vi "NetCDFLabviewDemo1.1.vi"(5 "NetCDF File:":path) -> ()   [LabVIEW 2016]
uses:
  DemoSubVIs/XControls/ArrayTree/ArrayTree.xctl
  DemoSubVIs/XControls/PairTable/PairTable.xctl
panel:
  in  "OK":bool
  in  "Tab Control":enum32{"Global ", "Detail"}(tab)
  out "Global Attributes":cluster{"c":string, "l":string}[](xcontrol)
  out "Attributes":cluster{"c":string, "l":string}[](xcontrol)
  out "var tree":T1(xcontrol)
  out "XY":cluster{dbl[], "value":dbl[]}[](graph) caption="H[0] 's graph"
  out "Text Variable":string caption="datetime[0](dump text)"
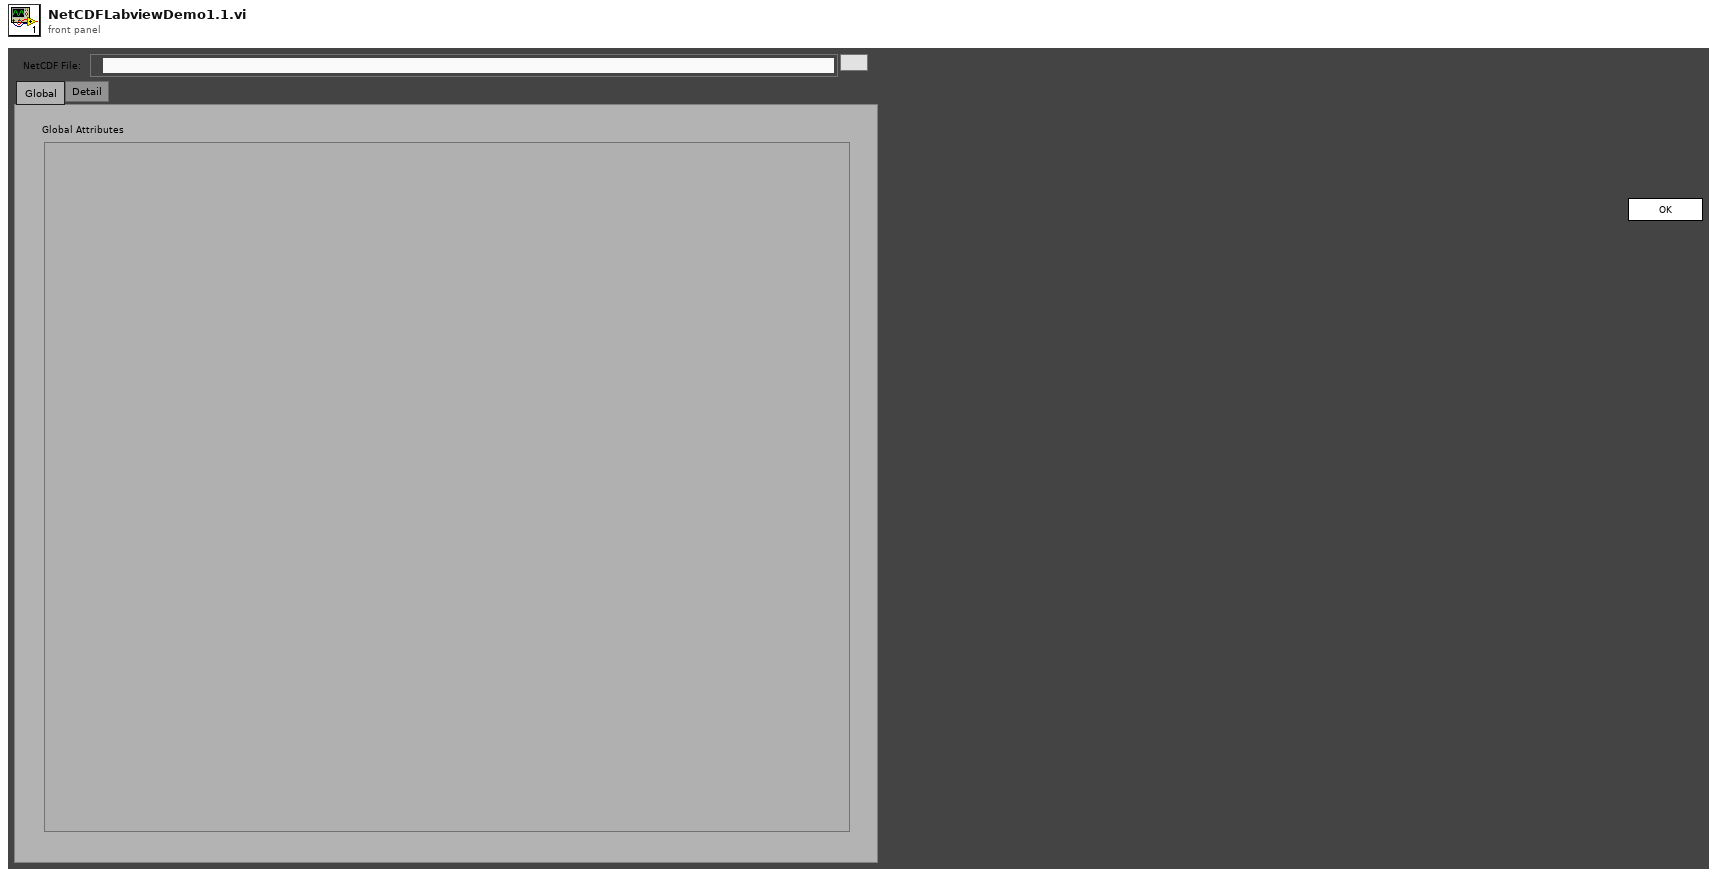
[diagram p1: front panel]
types:
  T1 = cluster{"TopLevelItemName":string, "ChildItemArr":cluster{"ChildDimName":string, "ChildDimSize":u64}[]}[]
  T2 = cluster{"TopLevelItemName":string, "ChildItemArr":cluster{"ChildDimName":string, "ChildDimSize":u64}[]}
  T3 = cluster{"numrecs":u64, "dims":cluster{"name":string, "size":u64}[], "attrs":cluster{"xsz":u64, "name":string, "nc_type":u16, "nelems":u64, "xvalue":string}[], "vars":cluster{"xsz":u64, "shape":u64[], "dsizes":u64[], "name":string, "dimids":u64[], "NC_attrarray":cluster{"xsz":u64, "name":string, "nc_type":u16, "nelems":u64, "xvalue":string}[], "nc_type":enum16{"NC_NAT", "NC_BYTE", "NC_CHAR", "NC_SHORT", "NC_INT", "NC_FLOAT", "NC_DOUBLE"}, "len":u64, "begin":u64}[]}
  T4 = cluster{"xsz":u64, "shape":u64[], "dsizes":u64[], "name":string, "dimids":u64[], "NC_attrarray":cluster{"xsz":u64, "name":string, "nc_type":u16, "nelems":u64, "xvalue":string}[], "nc_type":enum16{"NC_NAT", "NC_BYTE", "NC_CHAR", "NC_SHORT", "NC_INT", "NC_FLOAT", "NC_DOUBLE"}, "len":u64, "begin":u64}[]
  T5 = cluster{"xsz":u64, "shape":u64[], "dsizes":u64[], "name":string, "dimids":u64[], "NC_attrarray":cluster{"xsz":u64, "name":string, "nc_type":u16, "nelems":u64, "xvalue":string}[], "nc_type":enum16{"NC_NAT", "NC_BYTE", "NC_CHAR", "NC_SHORT", "NC_INT", "NC_FLOAT", "NC_DOUBLE"}, "len":u64, "begin":u64}
  T6 = enum32{"Invalid", "Standard", "Closed", "Hidden", "Minimized", "Maximized"}
  T7 = enum32{"invalid app kind", "Development System", "Run Time System", "Student Edition", "Embedded LabVIEW", "Evaluation", "Custom"}
  T8 = cluster{"Core":cluster{"Current VI Reference":refnum<vi>, "Close Panel on Exit?":bool}, "File Path":path, "file reference":refnum<k0>, "VarIndexArr":cluster{"TopLevelItemName":string, "ChildItemArr":cluster{"ChildDimName":string, "ChildDimSize":u64}[]}, "NC":cluster{"numrecs":u64, "dims":cluster{"name":string, "size":u64}[], "attrs":cluster{"xsz":u64, "name":string, "nc_type":u16, "nelems":u64, "xvalue":string}[], "vars":cluster{"xsz":u64, "shape":u64[], "dsizes":u64[], "name":string, "dimids":u64[], "NC_attrarray":cluster{"xsz":u64, "name":string, "nc_type":u16, "nelems":u64, "xvalue":string}[], "nc_type":enum16{"NC_NAT", "NC_BYTE", "NC_CHAR", "NC_SHORT", "NC_INT", "NC_FLOAT", "NC_DOUBLE"}, "len":u64, "begin":u64}[]}, "var-lowest-dim name pair":cluster{"name":string, "name":string}[]}
  T9 = cluster{"Current VI Reference":refnum<vi>, "Close Panel on Exit?":bool}
  T10 = cluster{"xsz":u64, "name":string, "nc_type":u16, "nelems":u64, "xvalue":string}[]
  T11 = cluster{"name":string, cluster{"name":string, "数值":u64}[]}[]
  T12 = enum16{"NC_NAT", "NC_BYTE", "NC_CHAR", "NC_SHORT", "NC_INT", "NC_FLOAT", "NC_DOUBLE"}
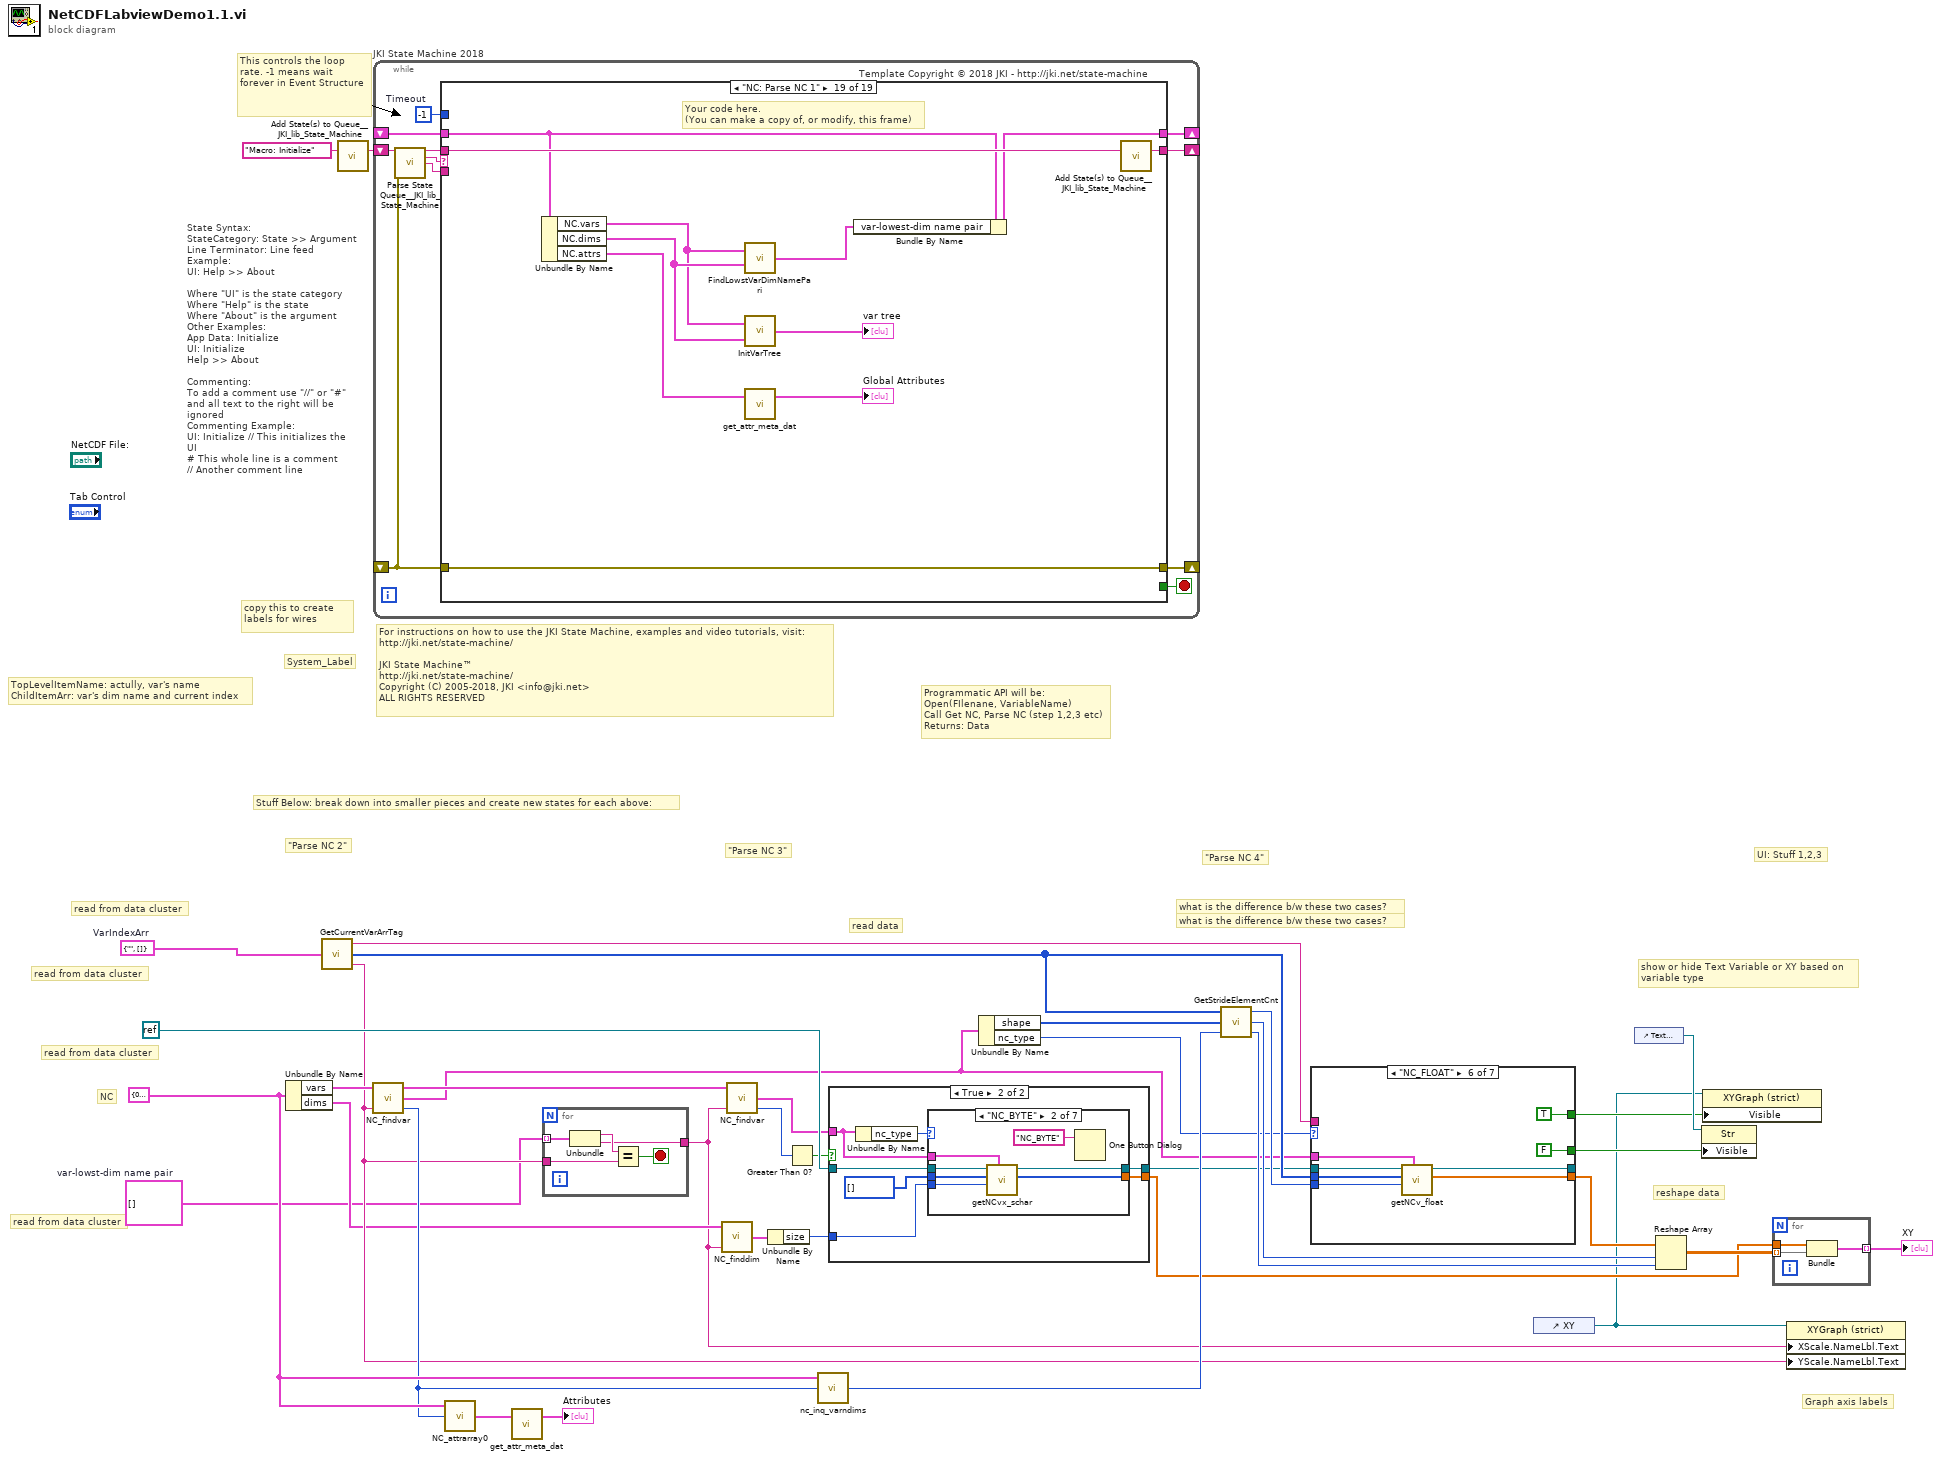
[diagram p0: block diagram]
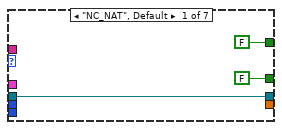
[diagram p2: hidden frame]
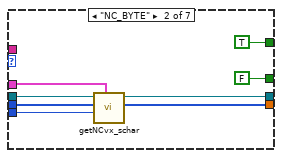
[diagram p3: hidden frame]
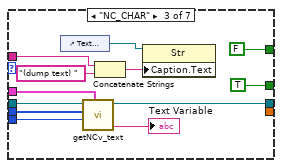
[diagram p4: hidden frame]
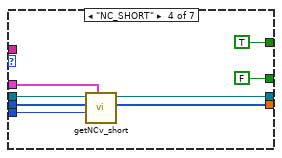
[diagram p5: hidden frame]
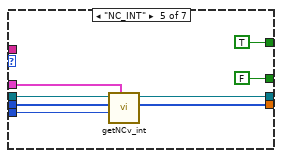
[diagram p6: hidden frame]
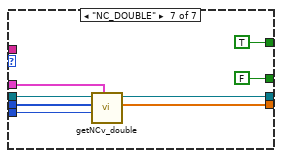
[diagram p7: hidden frame]
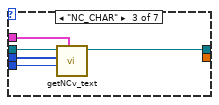
[diagram p10: hidden frame]
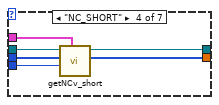
[diagram p11: hidden frame]
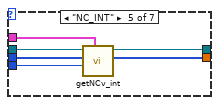
[diagram p12: hidden frame]
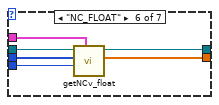
[diagram p13: hidden frame]
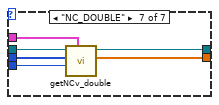
[diagram p14: hidden frame]
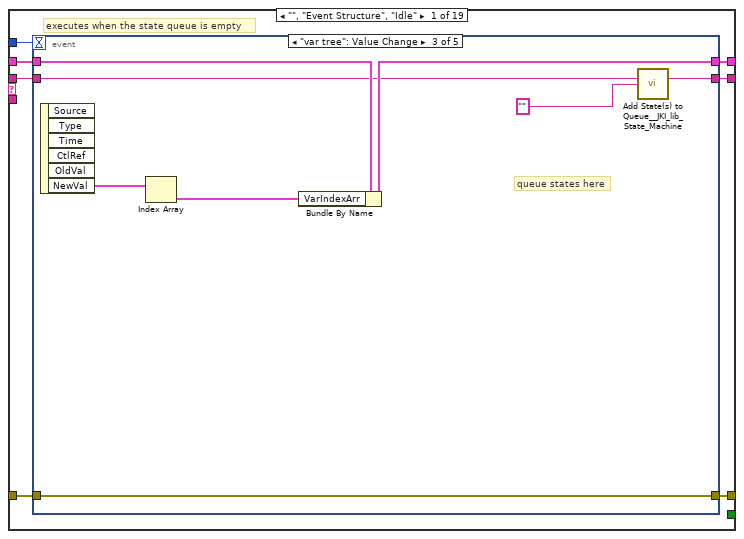
[diagram p15: hidden frame]
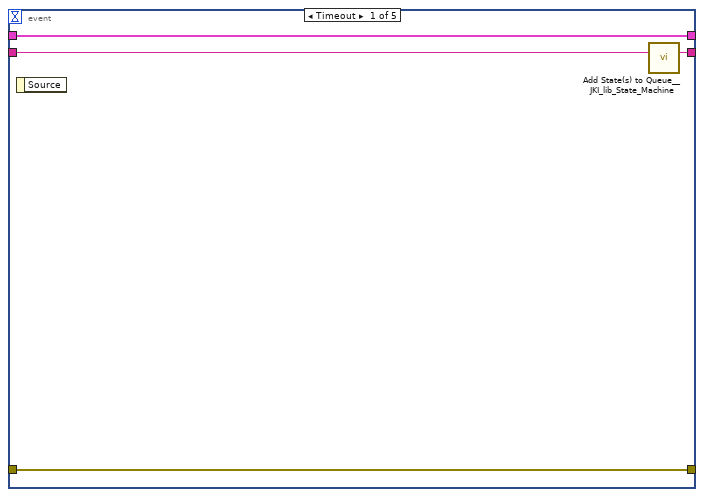
[diagram p16: hidden frame]
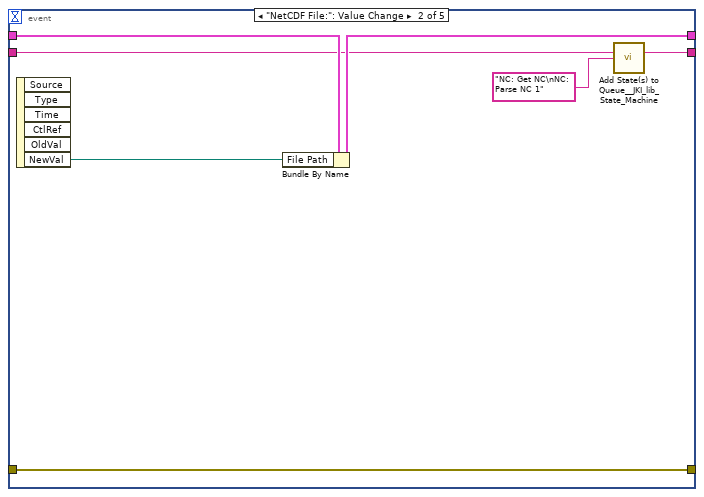
[diagram p17: hidden frame]
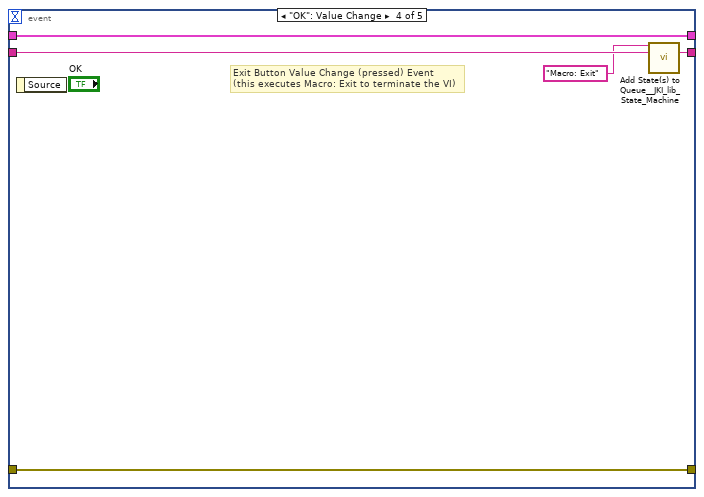
[diagram p18: hidden frame]
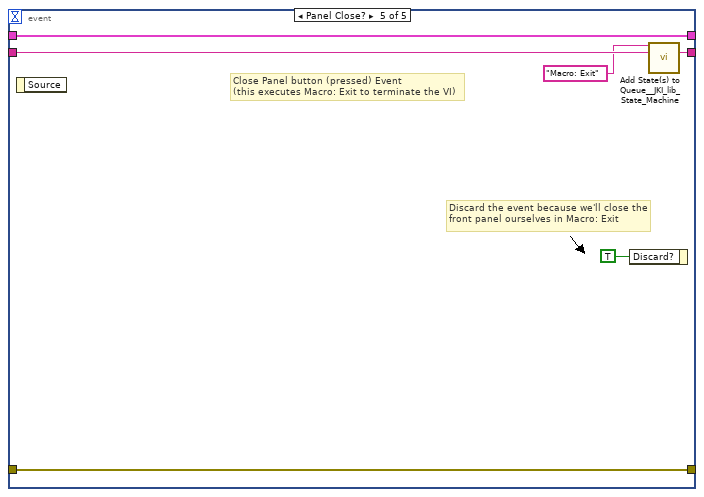
[diagram p19: hidden frame]
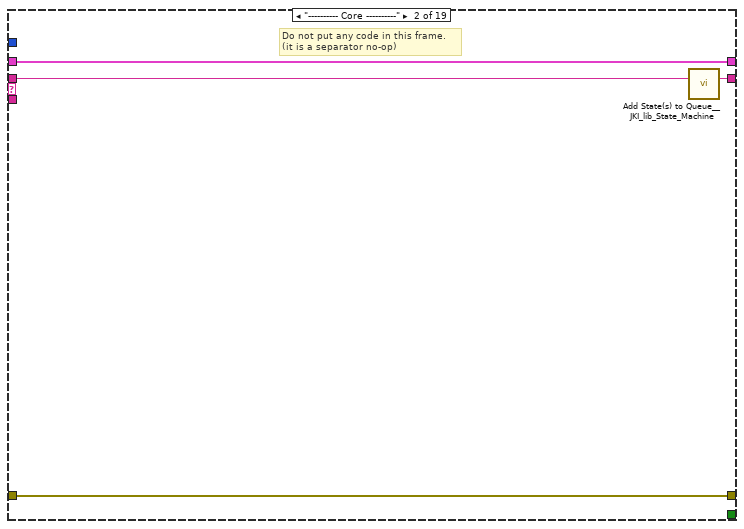
[diagram p20: hidden frame]
diagram:
  w4 = T2 {"TopLevelItemName"="", "ChildItemArr"=[]}  # VarIndexArr
  w2 = cluster{"name":string, "name":string}[] []  # var-lowst-dim name pair
  w34 = T3 {"numrecs"=0, "dims"=[], "attrs"=[], "vars"=[]} ("NC")
  # "Stuff Below: break down into smaller pieces and create new states for each above:"
  # "\"Parse NC 4\""
  # "\"Parse NC 3\""
  # "read from data cluster"
  # "read from data cluster"
  # "read data"
  # "Graph axis labels"
  # "UI: Stuff 1,2,3"
  # "\"Parse NC 2\""
  # "what is the difference b/w these two cases?"
  # "what is the difference b/w these two cases?"
  # "reshape data"
  # "show or hide Text Variable or XY based on\nvariable type"
  # "read from data cluster"
  # "read from data cluster"
  # "Programmatic API will be:\nOpen(FIlenane, VariableName)\nCall Get NC, Parse NC (step 1,2,3 etc)\nReturns: Data"
  # "For instructions on how to use the JKI State Machine, examples and video tutorials, visit:\nhttp://jki.net/state-machine/\n\nJKI State Machine™\nhttp://jki.net/state-machine/\nCopyright (C) 2005-2018, JKI <info@jki.net>\nALL RIGHTS RESERVED"
  # "State Syntax:\nStateCategory: State >> Argument\nLine Terminator: Line feed\nExample:\nUI: Help >> About\n\nWhere \"UI\" is the state category\nWhere \"Help\" is the state\nWhere \"About\" is the argument\nOther Examples:\nApp Data: Initialize\nUI: Initialize\nHelp >> About\n\nCommenting:\nTo add a comment use \"//\" or \"#\" and all text to the right will be ignored\nCommenting Example:\nUI: Initialize // This initializes the UI\n# This whole line is a comment\n// Another comment line"
  # "copy this to create labels for wires"
  # "This controls the loop rate. -1 means wait forever in Event Structure"
  # "System_Label"
  # "TopLevelItemName: actully, var's name\nChildItemArr: var's dim name and current index"
  # "NC"
  n1 = Unbundle By Name(w34) -> ("vars"=w14:T4, "dims"=w11:cluster{"name":string, "size":u64}[])
  n2 = call "GetCurrentVarArrTag.vi"("VarIndexArr"=w4) -> ("CurrentArrayTag"=w16:string, "IndexTagArr"=w18:u64[], "TopLevelItemName"=w13:string)
  n3 = call <vilib>:"Add State(s) to Queue__JKI_lib_State_Machine.vi"("State(s) in (\"\")"="Macro: Initialize") -> ("States Out"=w36:string)  [unwired: 14 in]
  n4 = call "NC_findvar.vi"("name"=w13, "NC_vararray"=w14) -> ("varid"=w29:i32, "NC_var"=w9:T5, "NC_vararray  out"=w12:T4)  [unwired: 1 out]
  n5 = while "JKI State Machine 2018" {
    shift-right: [w41] -> _
    shift-left: _ -> [w40]
    shift-right: [w44] -> _
    shift-left: _ -> [w38]
    shift-right: [w43] -> _
    shift-left: w36 -> [w45]
    stop <- w42 stop-if-true
    w39 = -1  # Timeout
    # "Template Copyright © 2018 JKI - http://jki.net/state-machine"
    n6 = call <vilib>:"Parse State Queue__JKI_lib_State_Machine.vi"("State Queue"=w45, "Error In (no error)"=w38) -> ("Remaining States"=w47:string, "Current State"=w48:string, "Arguments"=w46:string)  [unwired: 11 in]
    n7 = case shown="\"NC: Parse NC 1\"" w48 {
      selector: w48 -> [_ _ w90 _ _ _ _ _ _ _ _ _ _ _ _ _ _ _ _]
      tunnel: w47 -> [w55 w89 w94 w113 w119 w124 w128 w138 w146 w150 w154 w160 w171 w240 w245 w255 w259 w268 w279]
      tunnel: w46 -> [_ _ _ _ _ _ _ _ _ _ _ w155 w165 _ _ _ _ _ _]
      tunnel: w40 -> [w53 w86 w92 w106 w116 w122 w125 _ w142 w147 w152 w158 w167 w237 w242 w252 w256 w261 w270]
      tunnel: [w52 w87 w96 w110 errorcluster {"status"=FALSE, "code"=0, "source"=""} ("error out") w121 w126 w135 w143 w148 w151 w156 w168 w238 w243 w253 w257 w264 w277] -> w44
      tunnel: w38 -> [w51 w87 w95 w110 w115 w121 w126 w135 w140 w148 w151 w157 w169 w238 w243 w253 w257 w265 w277]
      tunnel: [w54 w88 w93 w112 w118 w123 w127 w137 w145 w149 w153 w159 w170 w239 w244 w254 w258 w267 w278] -> w43
      tunnel: [_ _ _ _ _ TRUE _ _ _ _ _ _ _ _ _ _ _ _ _] -> w42
      tunnel: [w50 w86 w92 w111 w116 w122 w125 w136 w142 w147 w152 w158 w167 w237 w242 w252 w256 w260 w269] -> w41
      tunnel: w39 -> [w49 _ _ _ _ _ _ _ _ _ _ _ _ _ _ _ _ _ _]
      frame "", "Event Structure", "Idle" {
        # "executes when the state queue is empty"
        n8 = event shown="[2] \"var tree\": Value Change" {
          selector: _ -> [_ _ _ _ _]
          dyn-events: _ -> [_ _ _ _ _]
          timeout: w49 -> [_ _ _ _ _]
          tunnel: w55 -> [w59 w61 w70 w79 w85]
          tunnel: [w58 w60 w69 w78 w84] -> w54
          tunnel: w53 -> [w56 w65 w73 w76 w82]
          tunnel: [w57 w66 w74 w77 w83] -> w52
          tunnel: w51 -> [w57 w66 w74 w77 w83]
          tunnel: [w56 w64 w72 w76 w82] -> w50
          event Timeout {
            n9 = event-data() -> ()  [unwired: 1 in, 1 out]
            n10 = call <vilib>:"Add State(s) to Queue__JKI_lib_State_Machine.vi"("State(s) in (\"\")"=w59) -> ("States Out"=w58:string)  [unwired: 14 in]
          }
          event "NetCDF File:": Value Change {
            n11 = event-data() -> ("NewVal"=w63:path)  [unwired: 1 in, 5 out]
            n12 = Bundle By Name(cluster=w65, "File Path"=w63) -> (w64:T8)
            n13 = call <vilib>:"Add State(s) to Queue__JKI_lib_State_Machine.vi"("State(s) in (\"\")"=w61, "State(s) at Back (\"\")"="NC: Get NC\nNC: Parse NC 1" ("State(s) at Back (\"\")")) -> ("States Out"=w60:string)  [unwired: 13 in]
          }
          event "var tree": Value Change {
            # "queue states here"
            n14 = event-data() -> ("NewVal"=w68:T1)  [unwired: 1 in, 5 out]
            n15 = Index Array(array=w68) -> (element=w67:T2)  [unwired: 1 in]
            n16 = Bundle By Name(cluster=w73, "VarIndexArr"=w67) -> (w72:T8)
            n17 = call <vilib>:"Add State(s) to Queue__JKI_lib_State_Machine.vi"("State(s) in (\"\")"=w70, "State(s) at Back (\"\")"="" ("State(s) at Back (\"\")")) -> ("States Out"=w69:string)  [unwired: 13 in]
          }
          event "OK": Value Change {
            # "Exit Button Value Change (pressed) Event\n(this executes Macro: Exit to terminate the VI)"
            n18 = event-data() -> ()  [unwired: 1 in, 1 out]
            n19 = call <vilib>:"Add State(s) to Queue__JKI_lib_State_Machine.vi"("State(s) in Front (\"\")"="Macro: Exit", "State(s) in (\"\")"=w79) -> ("States Out"=w78:string)  [unwired: 13 in]
          }
          event Panel Close? {
            # "Discard the event because we'll close the front panel ourselves in Macro: Exit"
            # "Close Panel button (pressed) Event\n(this executes Macro: Exit to terminate the VI)"
            n20 = event-data() -> ()  [unwired: 1 in, 1 out]
            n21 = event-data("Discard?"=TRUE) -> ()  [unwired: 1 in, 1 out]
            n22 = call <vilib>:"Add State(s) to Queue__JKI_lib_State_Machine.vi"("State(s) in Front (\"\")"="Macro: Exit", "State(s) in (\"\")"=w85) -> ("States Out"=w84:string)  [unwired: 13 in]
          }
        }
      }
      frame "---------- Core ----------" {
        # "Do not put any code in this frame.\n(it is a separator no-op)"
        n23 = call <vilib>:"Add State(s) to Queue__JKI_lib_State_Machine.vi"("State(s) in (\"\")"=w89) -> ("States Out"=w88:string)  [unwired: 14 in]
      }
      frame Default {
        w99 = 42 items=["No error", "Argument error", "Memory is full", "Out of zone", "End of file", "File already open", "Generic file I/O error", "File not found", "File permission error", "Disk is full", "Duplicate path", "Too many files open", "System feature not enabled", "Resource file not found", "Cannot add resource", "Resource not found", "Image not found", "Image memory error", "Pen does not exist", "Config type invalid", "Config token not found", "Config parse error", "Config memory error", "Bad external code format", "Bad external code offset", "External code not present", "Null window", "Destroy window error", "Null menu", "Print aborted", "Bad print record", "Print driver error", "Windows error during printing", "Memory error during printing", "Print dialog error", "Generic print error", "Invalid device refnum", "Device not found", "Device parameter error", "Device unit error", "Cannot open device", "Device call aborted", "Generic error", "Cancelled by user", "Object ID too low", "Object ID too high", "Object not in heap", "Unknown heap", "Unknown object (invalid DefProc)", "Unknown object (DefProc not in table)", "Message out of range", "Invalid (null) method", "Unknown message", "Manager call not supported", "Bad address", "Network operation in progress", "Network operation timed out", "Connection is busy", "Network attribute not supported", "Network error", "Address in use", "System out of memory", "Connection aborted", "Connection refused", "Not connected", "Already connected", "Connection closed", "Initialization error (interapplication manager)", "Bad occurrence", "Wait on unbound occurrence handler", "Occurrence queue overflow", "Datalog type conflict", "Unused", "Unrecognized type (interapplication manager)", "Memory corrupt", "Failed to make temporary DLL", "Old CIN version", "Drag socket not found", "Failed to load drop-object", "Failed to register OLE object", "Failed to release OLE object", "Format specifier type mismatch", "Unknown format specifier", "Too few format specifiers", "Too many format specifiers", "Scan failed", "Newer CIN version", "Error converting to variant", "Runtime menu error", "Password tampered", "Variant attribute not found", "Incompatible variant data type", "Event data is not available", "Event Store is not present", "Occurrence is not found", "Event Queue is not created", "Event info is not available", "Refnum passed is NULL", "Error retrieving Class GUID", "Error retrieving CoClass GUID", "Error retrieving TypeLib GUID.", "Bad built application magic bytes.", "Specific driver is different from the specific driver associated with the Logical Name.", "There is no session opened to the class driver.", "Max Error", "MAX - Error with config objects", "MAX - Error loading configuration", "MAX - Group not supported"]
        # "Current State"
        # "Do not delete, rename, or modify this frame.\n(this is used to capture unhandled states and typos)"
        # "Handle mistyped state name (developer tool)"
        n24 = Format Into String(format string="Software Exception: Unhandled State \"%s\"." ("message"), error in=w95, w90) -> (resulting string=w98:string, error out=w97:errorcluster)  [unwired: 1 in]
        n25 = call <vilib>:"Error Cluster From Error Code.vi"("show call chain? (False)"=TRUE, "error in (no error)"=w97, "error message (\"\")"=w98, "error code (0)"=w99) -> ("error out"=w96:errorcluster)  [unwired: 5 in]
        n26 = call <vilib>:"Add State(s) to Queue__JKI_lib_State_Machine.vi"("State(s) in (\"\")"=w94) -> ("States Out"=w93:string)  [unwired: 14 in]
      }
      frame "Initialize Core Data" {
        # "Do not delete, rename, or modify this frame.\n(this is used to determine panel behavior on exit)"
        # "originally closed?"
        # "exe?"
        # "If panel starts closed or is an EXE, then close it when we exit"
        n27 = property class="VI"() -> ("FP.State"=w103:T6)  [unwired: 2 in, 2 out]
        n28 = property class="App"() -> ("App.Kind"=w109:T7)  [unwired: 2 in, 2 out]
        n29 = control-ref of="Current VI Reference"() -> (w104:refnum<vi>)
        n30 = Equal?(x=w103, y=T6."Closed" ("Front Panel Window:State")) -> (x = y?=w101:bool)
        n31 = Equal?(x=w109, y=T7."Run Time System" ("Application:Kind")) -> (x = y?=w107:bool)
        n32 = Or(x=w101, y=w107) -> (x .or. y?=w105:bool)
        n33 = Bundle By Name(cluster=w106, "Core.Current VI Reference"=w104, "Core.Close Panel on Exit?"=w105) -> (w111:T8)
        n34 = call <vilib>:"Add State(s) to Queue__JKI_lib_State_Machine.vi"("State(s) in (\"\")"=w113) -> ("States Out"=w112:string)  [unwired: 14 in]
      }
      frame "Error Handler" {
        # "Unhandled Error -- Display it"
        # "Handle any errors here.\nYou can also output any states to clean-up after errors occur"
        # "Clear error"
        n35 = call <vilib>:"General Error Handler.vi"("error in (no error)"=w115) -> ()  [unwired: 10 in, 5 out]
        n36 = call <vilib>:"Add State(s) to Queue__JKI_lib_State_Machine.vi"("State(s) in Front (\"\")"="/* Post Error States", "State(s) in (\"\")"=w119) -> ("States Out"=w118:string)  [unwired: 13 in]
      }
      frame "Exit" {
        # "Do not put any code in this frame.\n(No errors that occur here will be handled.)"
        n37 = call <vilib>:"Add State(s) to Queue__JKI_lib_State_Machine.vi"("State(s) in (\"\")"=w124) -> ("States Out"=w123:string)  [unwired: 14 in]
      }
      frame "---------- Data ----------" {
        # "Do not put any code in this frame.\n(It is a separator no-op. You can make a copy of this frame to create a new Data frame)"
        n38 = call <vilib>:"Add State(s) to Queue__JKI_lib_State_Machine.vi"("State(s) in (\"\")"=w128) -> ("States Out"=w127:string)  [unwired: 14 in]
      }
      frame "Data: Initialize" {
        w129 = T2 {"TopLevelItemName"="", "ChildItemArr"=[]}  # VarIndexArr
        w130 = cluster{"name":string, "name":string}[] []  # var-lowest-dim name pair
        w131 = refnum<k0> refnum  # file reference
        w132 = path ""  # File Path
        w133 = T3 {"numrecs"=0, "dims"=[], "attrs"=[], "vars"=[]}  # NC
        w134 = T9 {"Current VI Reference"=refnum, "Close Panel on Exit?"=FALSE}  # Core
        # "Initialize the shift-register data, here.\n(data names are defined by what you wire into the bundle function)"
        n39 = Bundle("Core"=w134, "File Path"=w132, "file reference"=w131, "VarIndexArr"=w129, "NC"=w133, "var-lowest-dim name pair"=w130) -> (w136:T8)  [unwired: 1 in]
        n40 = call <vilib>:"Add State(s) to Queue__JKI_lib_State_Machine.vi"("State(s) in (\"\")"=w138) -> ("States Out"=w137:string)  [unwired: 14 in]
      }
      frame "Data: Cleanup" {
        # "Cleanup any data and references, here.\n(this is called automatically, by the Macro: Exit)"
        n41 = Unbundle By Name(w142) -> ("Core.Current VI Reference"=w144:refnum<vi>, "file reference"=w141:refnum<k0>)
        n42 = Close File(refnum=w141, error in=w140) -> (error out=w139:errorcluster)  [unwired: 1 out]
        n43 = Close Reference(reference=w144, error in (no error)=w139) -> (error out=w143:errorcluster)
        n44 = call <vilib>:"Add State(s) to Queue__JKI_lib_State_Machine.vi"("State(s) in (\"\")"=w146) -> ("States Out"=w145:string)  [unwired: 14 in]
      }
      frame "---------- UI ----------" {
        # "Do not put any code in this frame.\n(It is a separator no-op. You can make a copy of this frame to create a new UI frame)"
        n45 = call <vilib>:"Add State(s) to Queue__JKI_lib_State_Machine.vi"("State(s) in (\"\")"=w150) -> ("States Out"=w149:string)  [unwired: 14 in]
      }
      frame "UI: Initialize" {
        # "Initialize the User Interface, here.\n(this is called automatically, by the Macro: Init)"
        n46 = call <vilib>:"Add State(s) to Queue__JKI_lib_State_Machine.vi"("State(s) in (\"\")"=w154) -> ("States Out"=w153:string)  [unwired: 14 in]
      }
      frame "UI: Cursor Set" {
        # "Argument"
        # "Set and Unset Cursor Busy.\n(Usage: \"UI: Cursor Set >> Busy|Idle\")"
        n47 = case shown="\"Idle\", Default" w155 {
          tunnel: w157 -> [w162 w164]
          tunnel: [w161 w163] -> w156
          frame "Idle", Default {
            n48 = call <vilib>:"Unset Busy.vi"("error in (no error)"=w162) -> ("error out"=w161:errorcluster)  [unwired: 10 in]
          }
          frame "Busy" {
            n49 = call <vilib>:"Set Busy.vi"("error in (no error)"=w164) -> ("error out"=w163:errorcluster)  [unwired: 9 in, 1 out]
          }
        }
        n50 = call <vilib>:"Add State(s) to Queue__JKI_lib_State_Machine.vi"("State(s) in (\"\")"=w160) -> ("States Out"=w159:string)  [unwired: 14 in]
      }
      frame "UI: Front Panel State" {
        # "Argument"
        # "Set Front Panel Open or Closed\n(Usage: \"UI: Front Panel State >> Open|Close\")"
        n51 = Unbundle By Name(w167) -> ("Core.Current VI Reference"=w166:refnum<vi>)
        n52 = case shown="\"Minimize\", \"Minimized\"" w165 {
          tunnel: w169 -> [w177 w192 w203 w216 w229]
          tunnel: [w179 w193 w205 w218 w231] -> w168
          tunnel: w166 -> [w178 w190 w204 w217 w230]
          frame "Open", "Standard", Default {
            w172 = T6."Standard" ("State")
            n53 = property class="VI"(reference=w178, error in=w177) -> (reference out=w175:refnum<vi>, error out=w176:errorcluster, "FP.State"=w174:T6)
            n54 = Not Equal?(x=w174, y=w172) -> (x != y?=w173:bool)
            n55 = case shown="True" w173 {
              tunnel: [w183 w185] -> w179
              tunnel: w176 -> [w182 w185]
              tunnel: w175 -> [w181 _]
              tunnel: w172 -> [w180 _]
              frame True {
                n56 = invoke class="VI" method="FP.Open"(reference=w181, error in=w182, "Activate"=TRUE, "State"=w180) -> (error out=w183:errorcluster)  [unwired: 1 in, 4 out]
              }
              frame False {
              }
            }
          }
          frame "Close", "Closed" {
            n57 = property class="VI"(reference=w190, error in=w192) -> (reference out=w189:refnum<vi>, error out=w191:errorcluster, "FP.State"=w187:T6)
            n58 = Not Equal?(x=w187, y=T6."Closed" ("Front Panel Window:State")) -> (x != y?=w186:bool)
            n59 = case shown="True" w186 {
              tunnel: [w194 w197] -> w193
              tunnel: w191 -> [w194 w196]
              tunnel: w189 -> [_ w195]
              frame False {
              }
              frame True {
                n60 = invoke class="VI" method="FP.Close"(reference=w195, error in=w196) -> (error out=w197:errorcluster)  [unwired: 1 in, 2 out]
              }
            }
          }
          frame "Hidden", "Hide" {
            w198 = T6."Hidden" ("State")
            n61 = property class="VI"(reference=w204, error in=w203) -> (reference out=w201:refnum<vi>, error out=w202:errorcluster, "FP.State"=w200:T6)
            n62 = Not Equal?(x=w200, y=w198) -> (x != y?=w199:bool)
            n63 = case shown="True" w199 {
              tunnel: [w209 w210] -> w205
              tunnel: w202 -> [w208 w210]
              tunnel: w201 -> [w207 _]
              tunnel: w198 -> [w206 _]
              frame True {
                n64 = invoke class="VI" method="FP.Open"(reference=w207, error in=w208, "State"=w206) -> (error out=w209:errorcluster)  [unwired: 2 in, 4 out]
              }
              frame False {
              }
            }
          }
          frame "Minimize", "Minimized" {
            w211 = T6."Minimized" ("State")
            n65 = property class="VI"(reference=w217, error in=w216) -> (reference out=w214:refnum<vi>, error out=w215:errorcluster, "FP.State"=w213:T6)
            n66 = Not Equal?(x=w213, y=w211) -> (x != y?=w212:bool)
            n67 = case shown="True" w212 {
              tunnel: [w222 w223] -> w218
              tunnel: w215 -> [w221 w223]
              tunnel: w214 -> [w220 _]
              tunnel: w211 -> [w219 _]
              frame True {
                n68 = invoke class="VI" method="FP.Open"(reference=w220, error in=w221, "State"=w219) -> (error out=w222:errorcluster)  [unwired: 2 in, 4 out]
              }
              frame False {
              }
            }
          }
          frame "Maximize", "Maximized" {
            w224 = T6."Maximized" ("State")
            n69 = property class="VI"(reference=w230, error in=w229) -> (reference out=w227:refnum<vi>, error out=w228:errorcluster, "FP.State"=w226:T6)
            n70 = Not Equal?(x=w226, y=w224) -> (x != y?=w225:bool)
            n71 = case shown="True" w225 {
              tunnel: [w235 w236] -> w231
              tunnel: w228 -> [w234 w236]
              tunnel: w227 -> [w233 _]
              tunnel: w224 -> [w232 _]
              frame True {
                n72 = invoke class="VI" method="FP.Open"(reference=w233, error in=w234, "State"=w232) -> (error out=w235:errorcluster)  [unwired: 2 in, 4 out]
              }
              frame False {
              }
            }
          }
        }
        n73 = call <vilib>:"Add State(s) to Queue__JKI_lib_State_Machine.vi"("State(s) in (\"\")"=w171) -> ("States Out"=w170:string)  [unwired: 14 in]
      }
      frame "---------- Macro ----------" {
        # "Do not put any code in this frame.\n(It is a separator no-op. You can make a copy of this frame to create a new Macro frame)"
        n74 = call <vilib>:"Add State(s) to Queue__JKI_lib_State_Machine.vi"("State(s) in (\"\")"=w240) -> ("States Out"=w239:string)  [unwired: 14 in]
      }
      frame "Macro: Initialize" {
        w241 = "Data: Initialize\nInitialize Core Data\nUI: Initialize\nUI: Front Panel State >> Open"  # Data: Initialize Initialize Core Data UI: Initialize UI: Front Panel State >> Open
        # "Initialization Macro\n(This is called once, when the VI starts)"
        n75 = call <vilib>:"Add State(s) to Queue__JKI_lib_State_Machine.vi"("State(s) in Front (\"\")"=w241, "State(s) in (\"\")"=w245) -> ("States Out"=w244:string)  [unwired: 13 in]
      }
      frame "Macro: Exit" {
        # "Exit Macro\n(This is called once, when the VI exits)"
        n76 = Unbundle By Name(w252) -> ("Core.Close Panel on Exit?"=w251:bool)
        n77 = Select(t="UI: Front Panel State >> Close", s=w251, f="") -> (s? t:f=w248:string)
        n78 = call <vilib>:"Add State(s) to Queue__JKI_lib_State_Machine.vi"("State(s) in (\"\")"=w248, "State(s) at Back (\"\")"="Data: Cleanup\nExit") -> ("States Out"=w246:string)  [unwired: 13 in]
        n79 = call <vilib>:"Add State(s) to Queue__JKI_lib_State_Machine.vi"("State(s) in Front (\"\")"=w246, "State(s) in (\"\")"=w255) -> ("States Out"=w254:string)  [unwired: 13 in]
      }
      frame "---------- NC ----------" {
        # "Template Separator\n(You can make a copy of, or modify, this frame)"
        n80 = call <vilib>:"Add State(s) to Queue__JKI_lib_State_Machine.vi"("State(s) in (\"\")"=w259) -> ("States Out"=w258:string)  [unwired: 14 in]
      }
      frame "NC: Get NC" {
        # "Your code here.\n(You can make a copy of, or modify, this frame)"
        n81 = Unbundle By Name(w261) -> ("File Path"=w266:path)
        n82 = call "nc_get_NC.vi"("ErrorIn"=w265, "FilePath"=w266) -> ("ErrorOut"=w264:errorcluster, "NC"=w262:T3, "refnum out"=w263:refnum<file>)  [unwired: 1 out]
        n83 = Bundle By Name(cluster=w261, "file reference"=w263, "NC"=w262) -> (w260:T8)
        n84 = call <vilib>:"Add State(s) to Queue__JKI_lib_State_Machine.vi"("State(s) in (\"\")"=w268) -> ("States Out"=w267:string)  [unwired: 14 in]
      }
      frame "NC: Parse NC 1" {
        # "Your code here.\n(You can make a copy of, or modify, this frame)"
        n85 = Unbundle By Name(w270) -> ("NC.vars"=w273:T4, "NC.dims"=w274:cluster{"name":string, "size":u64}[], "NC.attrs"=w275:T10)
        n86 = call "FindLowstVarDimNamePari.vi"("dims"=w274, "vars"=w273) -> ("var-lowst-dim name pair"=w271:cluster{"name":string, "name":string}[])
        n87 = call "InitVarTree.vi"("dims"=w274, "vars"=w273) -> ("var tree"=→"var tree":T11)
        n88 = call "get_attr_meta_dat.vi"("NC_attrarray"=w275) -> ("NC_attr_meta_data_arr"=→"Global Attributes":cluster{"name":string, "xvalue":string}[])  [unwired: 1 in, 1 out]
        n89 = Bundle By Name(cluster=w270, "var-lowest-dim name pair"=w271) -> (w269:T8)
        n90 = call <vilib>:"Add State(s) to Queue__JKI_lib_State_Machine.vi"("State(s) in (\"\")"=w279) -> ("States Out"=w278:string)  [unwired: 14 in]
      }
    }
  }
  n91 = call "NC_attrarray0.vi"("varid"=w29, "NC"=w34) -> ("NC_attrarray"=w30:T10)  [unwired: 1 in, 2 out]
  n92 = call "get_attr_meta_dat.vi"("NC_attrarray"=w30) -> ("NC_attr_meta_data_arr"=→"Attributes":cluster{"name":string, "xvalue":string}[])  [unwired: 2 out]
  n93 = for {
    tunnel: w2 -> [w282] mode=indexing
    tunnel: w13 -> [w284]
    tunnel: [w280] -> w5
    stop <- w283 stop-if-true
    n94 = Unbundle(w282) -> ("name"=w281:string, "name"=w280:string)
    n95 = Equal?(x=w281, y=w284) -> (x = y?=w283:bool)
  }
  n96 = call "NC_finddim.vi"("name"=w5, "NC_dimarray"=w11) -> ("NC_dim"=w33:cluster{"name":string, "size":u64})  [unwired: 3 out]
  n97 = call "NC_findvar.vi"("name"=w5, "NC_vararray"=w12) -> ("varid"=w10:i32, "NC_var"=w31:T5)  [unwired: 2 out]
  n98 = Unbundle By Name(w33) -> ("size"=w32:u64)
  n99 = Greater Than 0?(x=w10) -> (x > 0?=w27:bool)
  n100 = call "nc_inq_varndims.vi"("varid"=w29, "NC"=w34) -> ("ndims"=w28:i32)  [unwired: 1 in, 2 out]
  n101 = case shown="True" w27 {
    tunnel: w32 -> [w286 w289]
    tunnel: w31 -> [_ w294]
    tunnel: [w285 w293] -> w3
    tunnel: [w287 w292] -> w7
    tunnel: refnum<k0> refnum -> [w287 w291]
    frame False {
      # "doesn't exist?"
      n102 = for {
        N: w286 -> [_]
        tunnel: [w288] -> w285 mode=indexing
        i -> [w288]
      }
    }
    frame True {
      n103 = Unbundle By Name(w294) -> ("nc_type"=w295:T12)
      n104 = case shown="\"NC_BYTE\"" w295 {
        tunnel: [_ w300 _ w313 w318 w323 w329] -> w293
        tunnel: w291 -> [w296 w302 w307 w314 w320 w326 w332]
        tunnel: w289 -> [_ w298 w306 w312 w319 w325 w331]
        tunnel: w294 -> [_ w301 w308 w311 w317 w324 w330]
        tunnel: [w296 w299 w305 w310 w316 w322 w328] -> w292
        tunnel: u64[] [] ("start") -> [_ w297 w304 w309 w315 w321 w327]
        frame "NC_NAT", Default {
        }
        frame "NC_BYTE" {
          n105 = call "getNCvx_schar.vi"("NC_var"=w301, "nelems"=w298, "start"=w297, "refnum"=w302) -> ("value"=w300:i8[], "refnum out"=w299:refnum<file>)  [unwired: 1 in, 2 out]
          n106 = One Button Dialog(message="NC_BYTE" ("消息")) -> ()  [unwired: 2 out]
        }
        frame "NC_CHAR" {
          n107 = call "getNCv_text.vi"("NC_var"=w308, "nelems"=w306, "start"=w304, "refnum"=w307) -> ("refnum out"=w305:refnum<file>)  [unwired: 1 in, 3 out]
        }
        frame "NC_SHORT" {
          n108 = call "getNCv_short.vi"("NC_var"=w311, "nelems"=w312, "start"=w309, "refnum"=w314) -> ("value"=w313:i16[], "refnum out"=w310:refnum<file>)  [unwired: 1 in, 2 out]
        }
        frame "NC_INT" {
          n109 = call "getNCv_int.vi"("NC_var"=w317, "nelems"=w319, "start"=w315, "refnum"=w320) -> ("value"=w318:i32[], "refnum out"=w316:refnum<file>)  [unwired: 1 in, 2 out]
        }
        frame "NC_FLOAT" {
          n110 = call "getNCv_float.vi"("NC_var"=w324, "nelems"=w325, "start"=w321, "refnum"=w326) -> ("value"=w323:sgl[], "refnum out"=w322:refnum<file>)  [unwired: 1 in, 2 out]
        }
        frame "NC_DOUBLE" {
          n111 = call "getNCv_double.vi"("NC_var"=w330, "nelems"=w331, "start"=w327, "refnum"=w332) -> ("value"=w329:dbl[], "refnum out"=w328:refnum<file>)  [unwired: 1 in, 2 out]
        }
      }
    }
  }
  n112 = Unbundle By Name(w9) -> ("shape"=w17:u64[], "nc_type"=w8:T12)
  n113 = call "GetStrideElementCnt.vi"("ndims"=w28, "shape"=w17, "CurrentIndex"=w18) -> ("shape[i-1]"=w26:u64, "shape[i-2]"=w25:u64, "strideElementCnt"=w19:u64)
  n114 = case shown="\"NC_FLOAT\"" w8 {
    tunnel: [_ w339 _ w362 w368 w375 w383] -> w6
    tunnel: w7 -> [w335 w343 w353 w363 w371 w379 w387]
    tunnel: w19 -> [_ w340 w351 w361 w369 w377 w385]
    tunnel: w16 -> [_ _ w347 _ _ _ _]
    tunnel: w18 -> [_ w341 w352 w359 w370 w378 w386]
    tunnel: w9 -> [_ w342 w354 w360 w367 w376 w384]
    tunnel: [w335 w338 w349 w358 w366 w374 w382] -> _
    tunnel: [FALSE ("可见") TRUE ("可见") FALSE ("可见") TRUE ("可见") TRUE ("可见") TRUE ("可见") TRUE ("可见")] -> w21
    tunnel: [FALSE ("可见") FALSE ("可见") TRUE ("可见") FALSE ("可见") FALSE ("可见") FALSE ("可见") FALSE ("可见")] -> w20
    frame "NC_NAT", Default {
    }
    frame "NC_BYTE" {
      n115 = call "getNCvx_schar.vi"("NC_var"=w342, "nelems"=w340, "start"=w341, "refnum"=w343) -> ("value"=w339:i8[], "refnum out"=w338:refnum<file>)  [unwired: 1 in, 2 out]
    }
    frame "NC_CHAR" {
      n116 = control-ref of="Text Variable"() -> (w355:refnum<vi>)
      n117 = call "getNCv_text.vi"("NC_var"=w354, "nelems"=w351, "start"=w352, "refnum"=w353) -> ("value"=→"Text Variable":string, "refnum out"=w349:refnum<file>)  [unwired: 1 in, 2 out]
      n118 = Concatenate Strings(w347, "(dump text) " ("字符串")) -> (w346:string)
      n119 = property class="Str"(reference=w355, "Caption.Text"=w346) -> ()  [unwired: 1 in, 2 out]
    }
    frame "NC_SHORT" {
      n120 = call "getNCv_short.vi"("NC_var"=w360, "nelems"=w361, "start"=w359, "refnum"=w363) -> ("value"=w362:i16[], "refnum out"=w358:refnum<file>)  [unwired: 1 in, 2 out]
    }
    frame "NC_INT" {
      n121 = call "getNCv_int.vi"("NC_var"=w367, "nelems"=w369, "start"=w370, "refnum"=w371) -> ("value"=w368:i32[], "refnum out"=w366:refnum<file>)  [unwired: 1 in, 2 out]
    }
    frame "NC_FLOAT" {
      n122 = call "getNCv_float.vi"("NC_var"=w376, "nelems"=w377, "start"=w378, "refnum"=w379) -> ("value"=w375:sgl[], "refnum out"=w374:refnum<file>)  [unwired: 1 in, 2 out]
    }
    frame "NC_DOUBLE" {
      n123 = call "getNCv_double.vi"("NC_var"=w384, "nelems"=w385, "start"=w386, "refnum"=w387) -> ("value"=w383:dbl[], "refnum out"=w382:refnum<file>)  [unwired: 1 in, 2 out]
    }
  }
  n124 = control-ref of="XY"() -> (w1:refnum<vi>)
  n125 = control-ref of="Text Variable"() -> (w22:refnum<vi>)
  n126 = Reshape Array(w6, w25, w26) -> (w24:dbl[][])
  n127 = property class="Str"(reference=w22, "Visible"=w20) -> ()  [unwired: 1 in, 2 out]
  n128 = property class="XYGraph (strict)"(reference=w1, "Visible"=w21) -> ()  [unwired: 1 in, 2 out]
  n129 = for {
    tunnel: w24 -> [w389] mode=indexing
    tunnel: [w390] -> w23 mode=indexing
    tunnel: w3 -> [w388]
    n130 = Bundle("value"=w388, "value"=w389) -> (w390:cluster{"value":dbl[], "value":dbl[]})  [unwired: 1 out]
  }
  "XY" <- w23
  n131 = property class="XYGraph (strict)"(reference=w1, "XScale.NameLbl.Text"=w5, "YScale.NameLbl.Text"=w13) -> ()  [unwired: 1 in, 2 out]
